vi "Pigeon2Setters.vi"   [LabVIEW 2023]
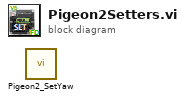
[diagram p0: block diagram]
diagram:
  n1 = call <vilib>:"Pigeon2_SetYaw.vi"() -> ()  [unwired: 12 in]
